vi "2048_init_board.vi"(9 "summon_ani":refnum<vi>, 10 "Arr Refnum in":refnum<vi>, 11 "Array in":refnum<vi>) -> (3 "Array out":i32[][](array[numeric]))   [LabVIEW 2021]
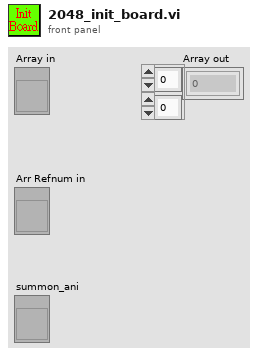
[diagram p1: front panel]
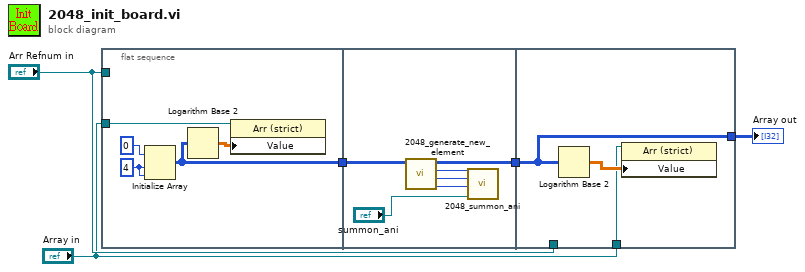
[diagram p0: block diagram]
diagram:
  n1 = flat-sequence {
    tunnel: [w7] -> w5
    tunnel: "Array in" -> [w6]
    tunnel: "Arr Refnum in" -> [_]
    tunnel: [w15] -> w4
    tunnel: w5 -> [w16]
    tunnel: w4 -> [w18]
    tunnel: [w18] -> w3
    tunnel: "Arr Refnum in" -> [_]
    tunnel: "Array in" -> [w17]
    frame #0 {
      w9 = 4 ("dimension size")
      n2 = Initialize Array(0 ("element"), w9, w9) -> (w7:i32[][])
      n3 = Logarithm Base 2(1:w7) -> (0:w8:dbl[][])
      n4 = property on="Property Node" class="Arr (strict)"(reference=w6, "Value"=w8) -> ()  [unwired: 1 in, 2 out]
    }
    frame #1 {
      n5 = call "2048_generate_new_element.vi"("Array in"=w16) -> ("c"=w12:u64, "r"=w13:u64, "element"=w14:i16, "Array out"=w15:i32[][])  [unwired: 7 in]
      n6 = call "2048_summon_ani.vi"("Array in"="summon_ani", "c"=w12, "r"=w13, "element"=w14) -> ()  [unwired: 8 in]
    }
    frame #2 {
      n7 = Logarithm Base 2(1:w18) -> (0:w19:dbl[][])
      n8 = property on="Property Node" class="Arr (strict)"(reference=w17, "Value"=w19) -> ()  [unwired: 1 in, 2 out]
    }
  }
  "Array out" <- w3
